vi "2.vi"() -> ()   [LabVIEW 2013]
panel:
  out "sorted array":dbl[](array[numeric])
  out "Array":dbl[](array[numeric])
  in  "Numeric":i32
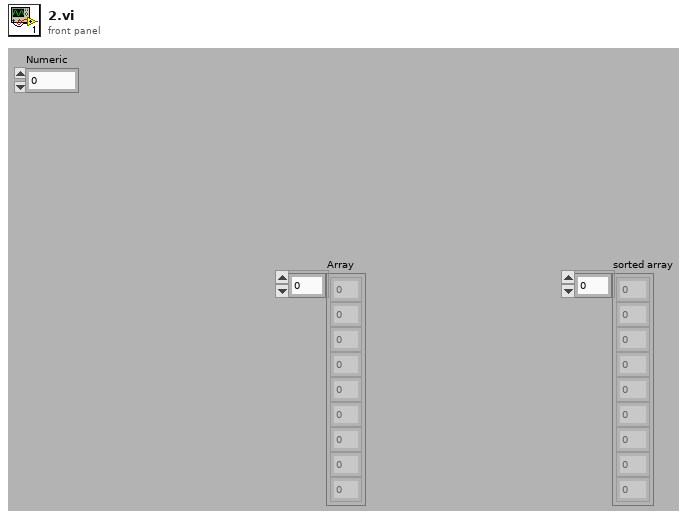
[diagram p1: front panel]
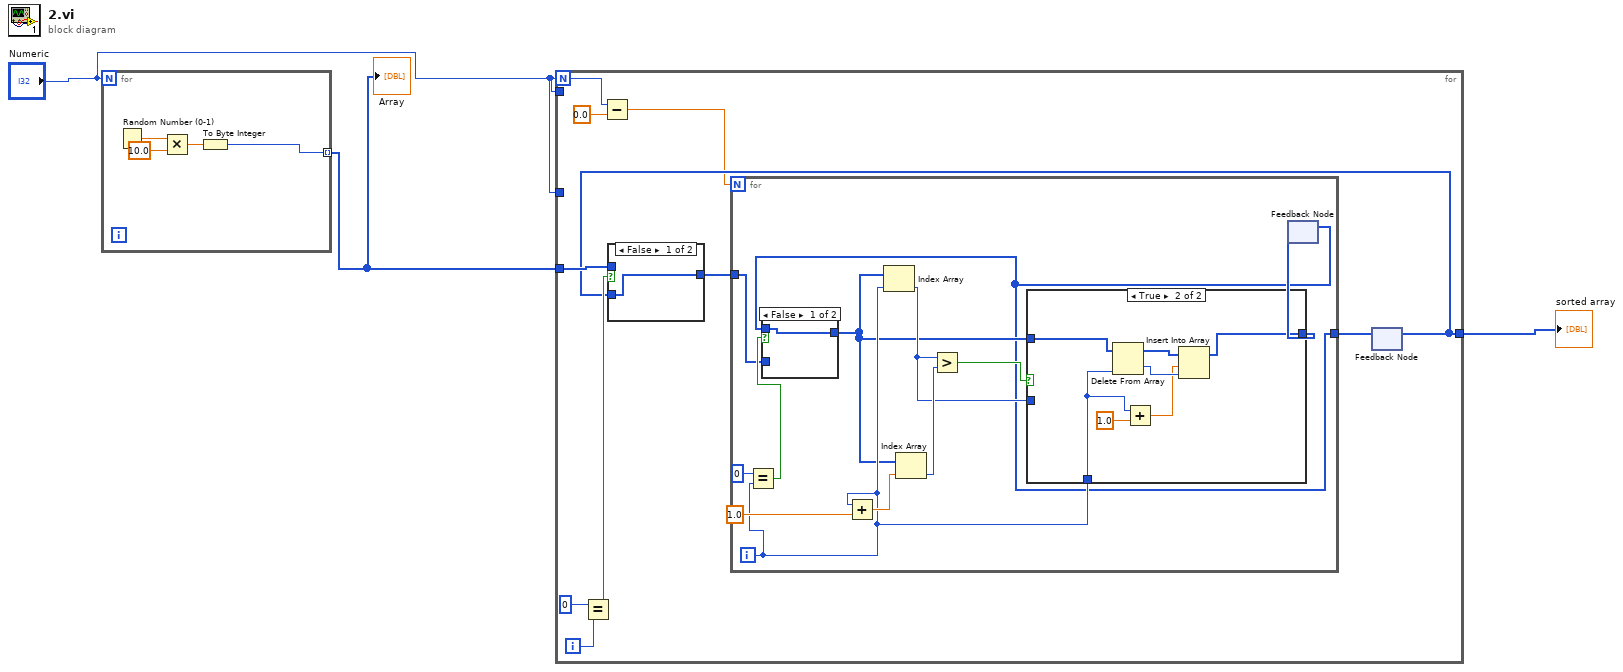
[diagram p0: block diagram]
diagram:
  n1 = for {
    N: "Numeric" -> [_]
    tunnel: [w4] -> w1 mode=indexing
    n2 = Random Number (0-1)() -> (number: 0 to 1=w7:dbl)
    n3 = Multiply(x=w7, y=10.0) -> (x*y=w5:dbl)
    n4 = To Byte Integer(number=w5) -> (8bit integer=w4:i8)
  }
  "Array" <- w1
  n5 = for {
    N: "Numeric" -> [w9]
    tunnel: w1 -> [w14]
    tunnel: "Numeric" -> [_]
    tunnel: [w11] -> w3
    tunnel: "Numeric" -> [_]
    i -> [w17]
    n6 = Equal?(x=0, y=w17) -> (x = y?=w15:bool)
    n7 = Subtract(x=w9, y=0.0) -> (x-y=w8:dbl)
    n8 = feedback #1() -> (w11:i8[])  [unwired: 1 in]
    n9 = case shown="False" w15 {
      tunnel: w14 -> [_ w19]
      tunnel: [w18 w19] -> w13
      tunnel: w11 -> [w18 _]
      frame False {
      }
      frame True {
      }
    }
    n10 = for {
      N: w8 -> [_]
      tunnel: w13 -> [w23]
      tunnel: [w20] -> w12
      i -> [w26]
      n11 = Equal?(x=0, y=w26) -> (x = y?=w24:bool)
      n12 = Add(x=w26, y=1.0) -> (x+y=w30:dbl)
      n13 = feedback #2() -> (w20:i8[])  [unwired: 1 in]
      n14 = case shown="False" w24 {
        tunnel: w23 -> [_ w33]
        tunnel: [w32 w33] -> w22
        tunnel: w20 -> [w32 _]
        frame False {
        }
        frame True {
        }
      }
      n15 = Index Array(array=w22, index=w26) -> (element=w27:i8)
      n16 = Index Array(array=w22, index=w30) -> (element=w29:i8)
      n17 = Greater?(x=w27, y=w29) -> (0:w28:bool)
      n18 = case shown="True" w28 {
        tunnel: w22 -> [w34 w41]
        tunnel: w27 -> [_ _]
        tunnel: w26 -> [_ w37]
        tunnel: [w34 w35] -> w21
        frame False {
        }
        frame True {
          n19 = Delete From Array(array=w41, index=w37) -> (deleted portion=w39:i8, array with subset deleted=w40:i8[])  [unwired: 1 in]
          n20 = Add(x=w37, y=1.0) -> (x+y=w36:dbl)
          n21 = Insert Into Array(array=w40, index=w36, new element=w39) -> (w35:i8[])
        }
      }
      n22 = feedback-in #2(w21) -> ()
    }
    n23 = feedback-in #1(w12) -> ()
  }
  "sorted array" <- w3
